vi "Register HTTP Handler.vi"(8 "error in (no error)":errorcluster, 10 "Handler":refnum<class "Handler.lvclass">, 11 "VolatusAPI in":refnum<class "VolatusAPI.lvclass">) -> (0 "error out":errorcluster, 3 "VolatusAPI out":refnum<class "VolatusAPI.lvclass">)   [LabVIEW 2020, in "Volatus.lvlib" / "VolatusAPI.lvclass"]
uses:
  VolatusAPI.lvclass
  lv-http-server/HTTP Server/Handler/Handler.lvclass
  VolatusAPI.lvclass/VolatusAPI.ctl
  lv-http-server/HTTP Server/Server/Add Connection Handler.vi
  lv-http-server/HTTP Server/Server/Add Request Handler.vi
  lv-http-server/HTTP Server/Server/Add Route Handler.vi
  lv-http-server/HTTP Server/Server/Add Controller Handler.vi
  lv-http-server/HTTP Server/Server/Add Controller.vi
  lv-http-server/HTTP Server/Server/Add Response Handler.vi
  lv-http-server/HTTP Server/Server/Add Complete Handler.vi
  lv-http-server/HTTP Server/Server/Add Exception Handler.vi
  lv-http-server/HTTP Server/Connection Handler/Connection Handler.lvclass
  lv-http-server/HTTP Server/Request Handler/Request Handler.lvclass
  lv-http-server/HTTP Server/Route Handler/Route Handler.lvclass
  lv-http-server/HTTP Server/Controller Handler/Controller Handler.lvclass
  lv-http-server/HTTP Server/Controller/Controller.lvclass
  lv-http-server/HTTP Server/Response Handler/Response Handler.lvclass
  lv-http-server/HTTP Server/Complete Handler/Complete Handler.lvclass
  lv-http-server/HTTP Server/Exception Handler/Exception Handler.lvclass
  lv-vecto/Vecto/Vecto/Vecto.lvclass
  lv-http-server/HTTP Server/Server/Server.lvclass
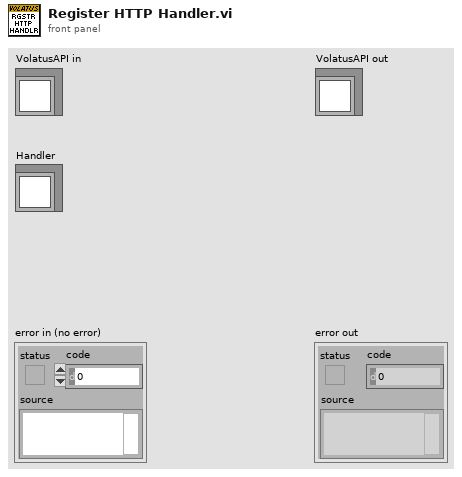
[diagram p1: front panel]
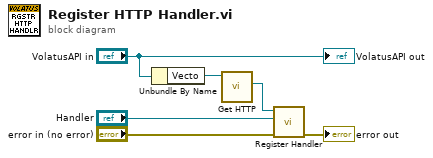
[diagram p0: block diagram]
diagram:
  n1 = Unbundle By Name("VolatusAPI in") -> ("Vecto"=w5:refnum<class "Vecto.lvclass">)
  n2 = call "Get HTTP.vi"("Vecto in"=w5) -> ("HTTP"=w4:refnum<class "Server.lvclass">)  [unwired: 8 in, 2 out]
  n3 = call "Register Handler.vi"("error in (no error)"="error in (no error)", "Handler"="Handler", "Server in"=w4) -> ("error out"=→"error out":errorcluster)  [unwired: 7 in, 1 out]
  "VolatusAPI out" <- "VolatusAPI in"
